vi "glb_引用.vi"() -> ()   [LabVIEW 2014]
panel:
  in  "WindowsMediaPlayer":refnum<vi>
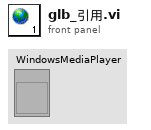
[diagram p1: front panel]
diagram:
